vi "题目6.vi"() -> ()   [LabVIEW 2017]
panel:
  out "平均值":dbl
  out "最小值":dbl
  out "最大值":dbl
  out "波形图":cluster{dbl[]}[](graph)
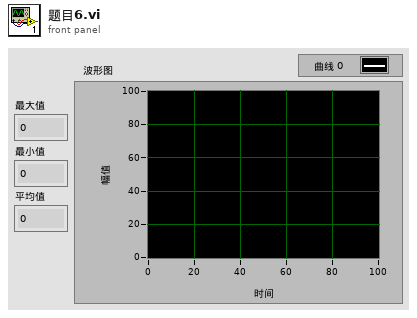
[diagram p1: front panel]
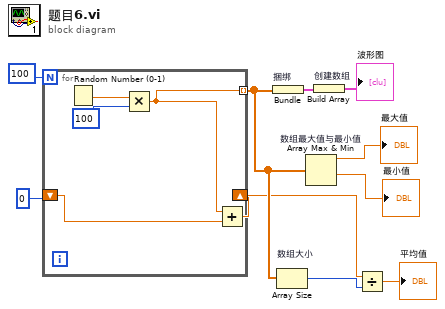
[diagram p0: block diagram]
diagram:
  n1 = for {
    N: 100 -> [_]
    shift-right: [w11] -> w2
    shift-left: 0 -> [w13]
    tunnel: [w12] -> w4 mode=indexing
    n2 = Random Number (0-1)() -> (number: 0 to 1=w15:dbl)
    n3 = Multiply(x=w15, y=100) -> (x*y=w12:dbl)
    n4 = Add(x=w12, y=w13) -> (x+y=w11:dbl)
  }
  n5 = Bundle "捆绑"(w4) -> (w8:cluster{dbl[]})  [unwired: 1 in]
  n6 = Array Size "数组大小"(array=w4) -> (size(s)=w3:i32)
  n7 = Array Max & Min "数组最大值与最小值"(array=w4) -> (max value=→"最大值":dbl, min value=→"最小值":dbl)  [unwired: 2 out]
  n8 = Build Array "创建数组"(w8) -> (→"波形图":cluster{dbl[]}[])
  n9 = Divide(x=w2, y=w3) -> (x/y=→"平均值":dbl)
